vi "Deadband.vi"() -> ()   [LabVIEW 2017]
panel:
  in  "+- Bounds":dbl=0.3 format="%#_13g"
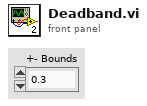
[diagram p1: front panel]
types:
  T1 = typedef "WPI_JoystickDevRef.ctl" = cluster{"Device":T2}
  T2 = typedef "WPI_JoystickDeviceEnum.ctl" = enum16{"USB 0", "USB 1", "USB 2", "USB 3", "USB 4", "USB 5"}
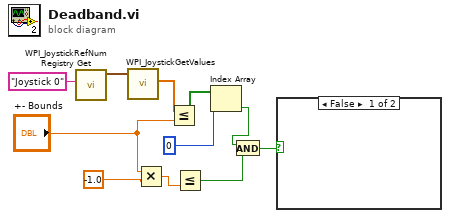
[diagram p0: block diagram]
diagram:
  n1 = call <vilib>:"WPI_JoystickRefNum Registry Get.vi"("refnum name"="Joystick 0") -> ("JoystickDevRef"=w6:T1)  [unwired: 9 in, 1 out]
  n2 = call <vilib>:"WPI_JoystickGetValues.vi"("JoystickDevRef"=w6) -> ("Axes"=w5:dbl[])  [unwired: 6 in, 4 out]
  n3 = Multiply(x="+- Bounds", y=-1.0) -> (x*y=w8:dbl)
  n4 = Less Or Equal?(x=w5, y="+- Bounds") -> (x <= y?=w4:bool[])
  n5 = Less Or Equal?(y=w8) -> (x <= y?=w7:bool)  [unwired: 1 in]
  n6 = Index Array(array=w4, index=0) -> (element=w3:bool)
  n7 = And(x=w3, y=w7) -> (x .and. y?=w1:bool)
  n8 = case shown="False" w1 {
    frame False {
    }
    frame True {
    }
  }
